vi "Platform Name.vi"(8 "error in (no error)":errorcluster, 11 "DeployTarget in":refnum<class "DeployTarget.lvclass">) -> (0 "error out":errorcluster, 2 "Platform Name":string, 3 "DeployTarget out":refnum<class "DeployTarget.lvclass">)   [LabVIEW 2020, in "PicoG-Core.lvlib" / "DeployTarget.lvclass"]
uses:
  DeployTarget.lvclass
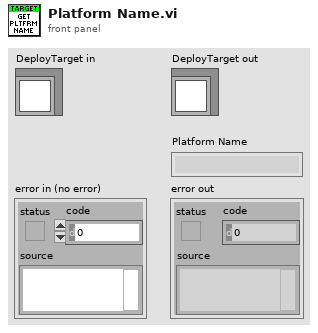
[diagram p1: front panel]
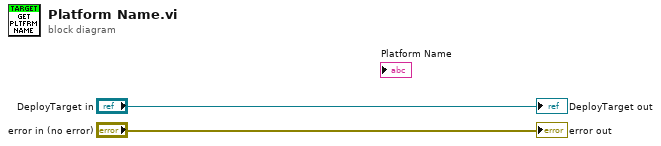
[diagram p0: block diagram]
diagram:
  "error out" <- "error in (no error)"
  "DeployTarget out" <- "DeployTarget in"
